vi "LoginUser.vi"(8 "error in (no error)":errorcluster, 9 "LastUserName":string, 10 "IsInitialLogin":bool, 11 "Sequence Context In":refnum<k7>) -> (0 "error out":errorcluster)   [LabVIEW 2020]
doc: "This is the top level VI called by the FrontEndCallbacks.seq file to launch and manage the login process in TestStand. To use this VI instead of the default CVI code to manage the login dialog, open the FrontEndCallbacks sequence (<TestStand Public>\\Components\\Callbacks\\Station\\StationCallbacks.seq), set the first two steps to \"skip\" and the last two to normal in run mode. Note: this code differs from the CVI version in that The users are selected by a ring control, and must be chosen; names cannot be manually typed"
panel:
  out "Sequence Context Out":refnum<k7>
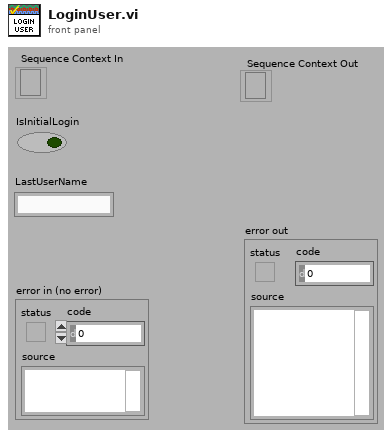
[diagram p1: front panel]
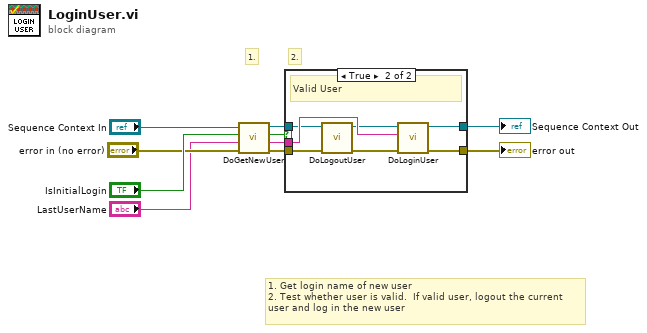
[diagram p0: block diagram]
diagram:
  # "1. Get login name of new user\n2. Test whether user is valid.  If valid user, logout the current user and log in the new user"
  # "1."
  # "2."
  n1 = call "DoGetNewUser.vi"("error in (no error)"="error in (no error)", "LastUserName"="LastUserName", "IsInitialLogin"="IsInitialLogin", "Sequence Context In"="Sequence Context In") -> ("error out"=w7:errorcluster, "LoginName"=w5:string, "isValidUser"=w8:bool, "Sequence Context Out"=w2:refnum<k7>)  [unwired: 3 in]
  n2 = case shown="True" w8 {
    tunnel: w2 -> [w12 w15]
    tunnel: w7 -> [w11 w19]
    tunnel: [w12 w18] -> w4
    tunnel: [w11 w17] -> w1
    tunnel: w5 -> [_ w16]
    frame False {
      # "Invalid User"
    }
    frame True {
      # "Valid User"
      n3 = call "DoLogoutUser.vi"("error in (no error)"=w19, "Sequence Context In"=w15) -> ("error out"=w14:errorcluster, "Sequence Context Out"=w13:refnum<k7>)  [unwired: 6 in]
      n4 = call "DoLoginUser.vi"("error in (no error)"=w14, "LoginName"=w16, "Sequence Context In"=w13) -> ("error out"=w17:errorcluster, "Sequence Context Out"=w18:refnum<k7>)  [unwired: 5 in]
    }
  }
  "error out" <- w1
  "Sequence Context Out" <- w4
